vi "Set Attenuation.vi"(8 "error in (no error)":errorcluster, 10 "Attenuation (dB)":dbl, 11 "Device ID in":i32) -> (0 "error out":errorcluster, 3 "Device ID out":i32)   [LabVIEW 2013, in "Vaunix LDA.lvlib"]
doc: "VNX_ATTEN_API LVSTATUS fnLDA_SetAttenuation(DEVID deviceID, int attenuation)\n\nThis function is used to set the attenuation level of the programmable attenuator. \n\nNote: The VI converts to what the function requires from Engineering units of dB.\n\nThe attenuation setting is encoded as an integer where each increment represents .25db of attenuation. The encoding is: attenuation * .25db = Attenuation in db\n\nFor example, attenuation = 40 for 10db of attenuation, 2 for .5db of attenuation (the minimum resolution of the LDA-102 and LDA-602 series hardware), and 252 for 63db attenuation."
uses:
  Vaunix LDA.lvlib
  VNX_atten.dll
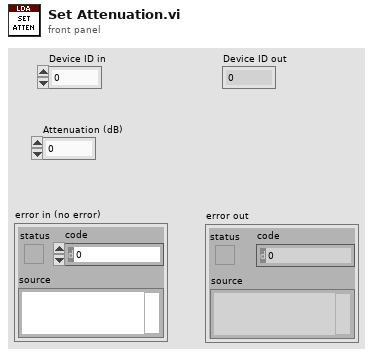
[diagram p1: front panel]
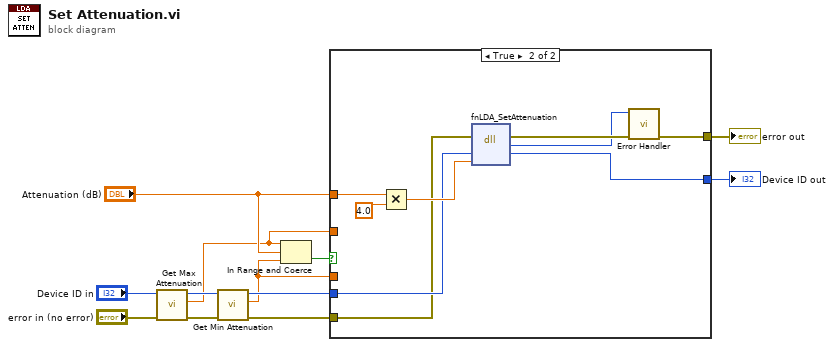
[diagram p0: block diagram]
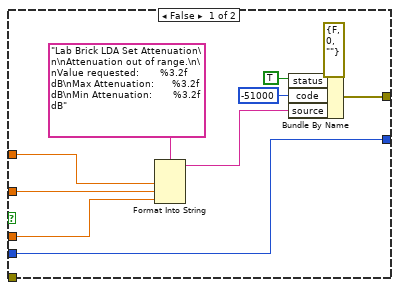
[diagram p2: hidden frame]
diagram:
  n1 = call "Get Max Attenuation.vi"("error in (no error)"="error in (no error)", "Device ID in"="Device ID in") -> ("error out"=w7:errorcluster, "Max Attenuation (dB)"=w1:dbl, "Device ID out"=w8:i32)  [unwired: 7 in]
  n2 = call "Get Min Attenuation.vi"("error in (no error)"=w7, "Device ID in"=w8) -> ("error out"=w5:errorcluster, "Min Attenuation (dB)"=w3:dbl, "Device ID out"=w6:i32)  [unwired: 7 in]
  n3 = In Range and Coerce(upper limit=w1, x="Attenuation (dB)", lower limit=w3) -> (In Range?=w4:bool)  [unwired: 1 out]
  n4 = case shown="True" w4 {
    tunnel: [w13 w31] -> w12
    tunnel: [w20 w29] -> w11
    tunnel: "Attenuation (dB)" -> [w17 w27]
    tunnel: w6 -> [w13 w24]
    tunnel: w5 -> [_ w23]
    tunnel: w3 -> [w15 _]
    tunnel: w1 -> [w16 _]
    frame False {
      n5 = Format Into String(format string="Lab Brick LDA Set Attenuation\n\nAttenuation out of range.\n\nValue requested:       %3.2f dB\nMax Attenuation:      %3.2f dB\nMin Attenuation:       %3.2f dB", w17, w16, w15) -> (resulting string=w14:string)  [unwired: 2 in, 1 out]
      n6 = Bundle By Name(cluster=errorcluster {"status"=FALSE, "code"=0, "source"=""} ("error out"), "status"=TRUE, "code"=-51000, "source"=w14) -> (w20:errorcluster)
    }
    frame True {
      n7 = Multiply(x=w27, y=4.0) -> (x*y=w25:dbl)
      n8 = dll-call lib="C:/Documents and Settings/Bauerle/Bureau/Partage/FPGA_Batch_1_7_3_1/Batch_main Folder/host-subvis/RF_attenuator/VNX_atten.dll" fn="fnLDA_SetAttenuation"(error in=w23, "deviceID"=w24, "attenuation"=w25) -> (error out=w30:errorcluster, "Status"=w28:i32, "deviceID"=w31:i32)  [unwired: 3 in, 1 out]
      n9 = call "Error Handler.vi"("error in (no error)"=w30, "Status"=w28) -> ("error out"=w29:errorcluster)  [unwired: 9 in]
    }
  }
  "error out" <- w11
  "Device ID out" <- w12
